vi "Open Close Project Window__icon_lib_labview_project_api.vi"(8 "error in (no error)":errorcluster, 10 "Open Project Window":bool, 11 "Project Reference":refnum<vi>) -> (0 "error out":errorcluster, 3 "Project Reference Dup":refnum<vi>)   [LabVIEW 2016, in "LabVIEW Project API__icon_lib_labview_project_api.lvlib"]
doc: "Open or Close a Project Window\n\n<b>Author:</b> JG\n\n<b>ICON Technologies Pty Ltd</b>\nCopyright (C) 1990-2009\nAll Rights Reserved"
uses:
  LabVIEW Project API__icon_lib_labview_project_api.lvlib
panel:
  # "Output"
  # "Input"
  # "ICON Technologies Pty Ltd\nCopyright (C) 1990-2009\nAll Rights Reserved"
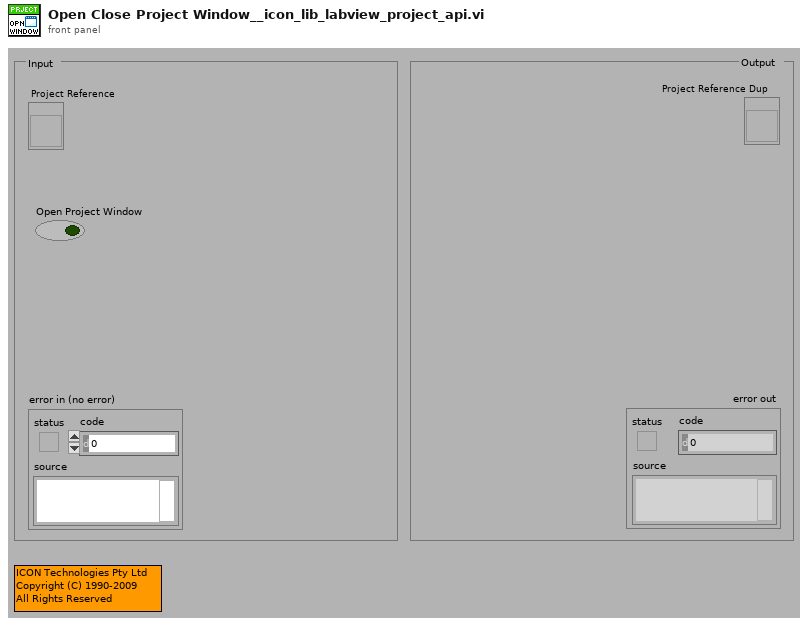
[diagram p1: front panel]
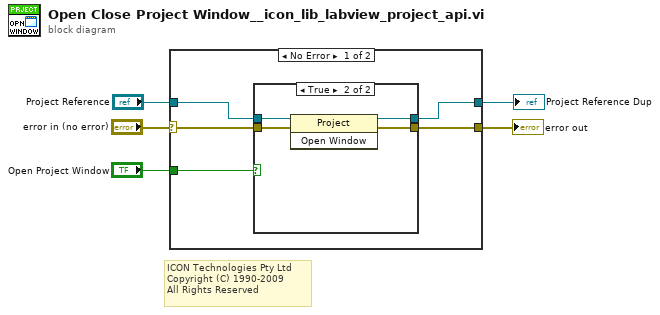
[diagram p0: block diagram]
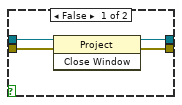
[diagram p2: hidden frame]
diagram:
  # "ICON Technologies Pty Ltd\nCopyright (C) 1990-2009\nAll Rights Reserved"
  n1 = case shown="No Error" "error in (no error)" {
    selector: "error in (no error)" -> [w7 w20]
    tunnel: [w8 w20] -> w4
    tunnel: "Project Reference" -> [w9 w19]
    tunnel: "Open Project Window" -> [w10 _]
    tunnel: [w6 w19] -> w1
    frame No Error {
      n2 = case shown="True" w10 {
        tunnel: w7 -> [w13 w18]
        tunnel: w9 -> [w14 w17]
        tunnel: [w12 w16] -> w6
        tunnel: [w11 w15] -> w8
        frame False {
          n3 = invoke class="Project" method="Close Window"(reference=w14, error in=w13) -> (reference out=w12:refnum<vi>, error out=w11:errorcluster)  [unwired: 1 in, 1 out]
        }
        frame True {
          n4 = invoke class="Project" method="Open Window"(reference=w17, error in=w18) -> (reference out=w16:refnum<vi>, error out=w15:errorcluster)  [unwired: 1 in, 1 out]
        }
      }
    }
    frame Error {
    }
  }
  "error out" <- w4
  "Project Reference Dup" <- w1
